vi "Replace Row In File.vi"(8 "error in":errorcluster, 9 "Index":i32, 10 "Insert Array":dbl[](array[numeric]), 11 "Path":path) -> (0 "error out":errorcluster)   [LabVIEW 2021]
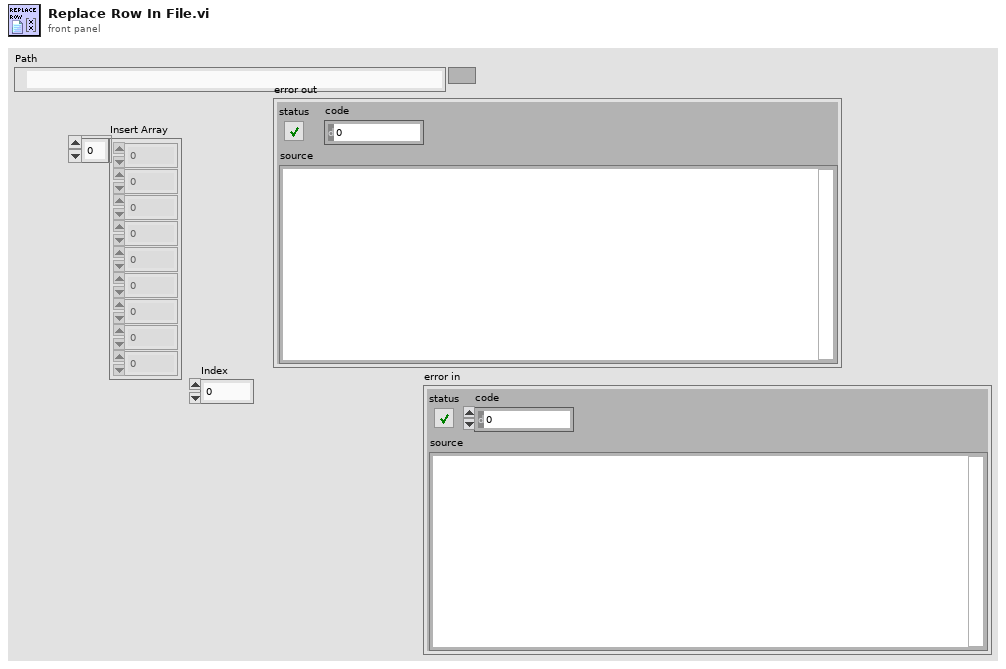
[diagram p1: front panel]
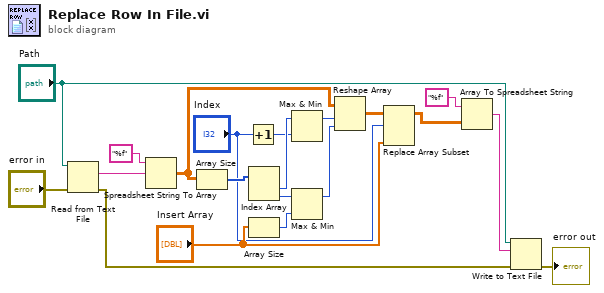
[diagram p0: block diagram]
diagram:
  n1 = Read from Text File(file (use dialog)="Path", error in="error in") -> (text=w17:string, error out=w1:errorcluster)  [unwired: 2 in, 2 out]
  n2 = Spreadsheet String To Array(format string="%f", spreadsheet string=w17) -> (array=w20:dbl[][])  [unwired: 2 in]
  n3 = Array Size(array=w20) -> (size(s)=w13:i32[])
  n4 = Increment(x="Index") -> (x+1=w9:i32)
  n5 = Index Array(array=w13) -> (element #1=w12:i32, element #2=w5:i32)  [unwired: 2 in]
  n6 = Array Size(array="Insert Array") -> (size(s)=w7:i32)
  n7 = Max & Min(x=w12, y=w9) -> (max(x,y)=w11:i32)  [unwired: 1 out]
  n8 = Max & Min(x=w5, y=w7) -> (max(x,y)=w6:i32)  [unwired: 1 out]
  n9 = Reshape Array(w20, w11, w6) -> (w10:dbl[][])
  n10 = Replace Array Subset(array=w10, new element="Insert Array", index (row)="Index") -> (w19:dbl[][])  [unwired: 1 in]
  n11 = Array To Spreadsheet String(array=w19, 3:"%f" ("format string")) -> (spreadsheet string=w16:string)  [unwired: 1 in]
  n12 = Write to Text File(file (use dialog)="Path", text=w16, error in=w1) -> (error out=→"error out":errorcluster)  [unwired: 1 in, 2 out]
